vi "Config Version.vi"(8 "error in (no error)":errorcluster, 11 "VolatusConfig in":refnum<class "VolatusConfig.lvclass">) -> (0 "error out":errorcluster, 2 "Config Version":string, 3 "VolatusConfig out":refnum<class "VolatusConfig.lvclass">)   [LabVIEW 2020, in "VolatusConfig.lvlib" / "VolatusConfig.lvclass"]
uses:
  VolatusConfig.lvclass
  VolatusConfig.lvclass/VolatusConfig.ctl
  lv-cdm/CDM-Config/Config Element/Config Element.lvclass
  Meta Name.ctl
  VolatusConfig.lvlib
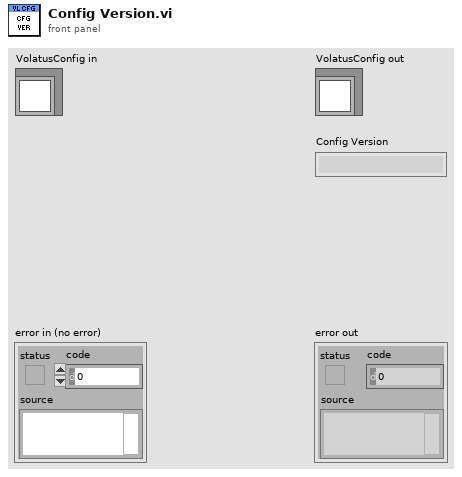
[diagram p1: front panel]
types:
  T1 = typedef "VolatusConfig.lvlib/Meta Name.ctl" = enum16{"VL_Type", "VL_Node_IP", "VL_Node_Type", "VL_Task_Type", "VL_Group_Type", "VL_Channel_Type", "VL_Channel_DataType", "VL_Config_Version"}
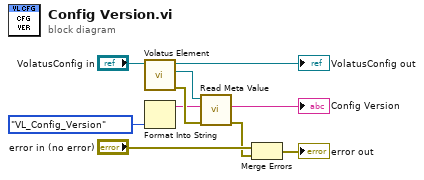
[diagram p0: block diagram]
diagram:
  n1 = call "Volatus Element.vi"("VolatusConfig in"="VolatusConfig in") -> ("error out"=w10:errorcluster, "Volatus Element"=w6:refnum<class "Config Element.lvclass">, "VolatusConfig out"=→"VolatusConfig out":refnum<class "VolatusConfig.lvclass">)  [unwired: 8 in]
  n2 = Format Into String(Meta_Name."VL_Config_Version" ("Meta Name")) -> (resulting string=w5:string)  [unwired: 3 in, 1 out]
  n3 = call "Read Meta Value.vi"("error in (no error)"=w10, "Meta Name"=w5, "Config Element in"=w6) -> ("error out"=w1:errorcluster, "Meta Value"=→"Config Version":string)  [unwired: 6 in, 1 out]
  n4 = Merge Errors("error in (no error)", w1) -> (→"error out":errorcluster)
